vi "Follow Tilt.vi"(4 "L/T":bool, 6 "deg":i16, 8 "In":u8[][](array[numeric])) -> (0 "Out":u8[][](array[numeric]))   [LabVIEW 2015]
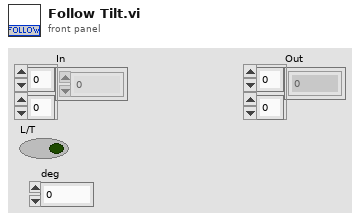
[diagram p1: front panel]
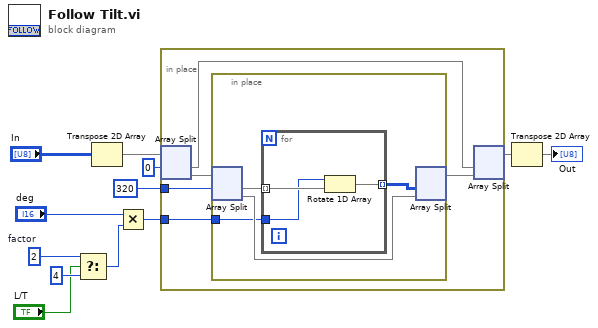
[diagram p0: block diagram]
diagram:
  w4 = i16 2  # factor
  n1 = Select(t=w4, s="L/T", f=i16 4) -> (s? t:f=w3:i16)
  n2 = Transpose 2D Array(2D array="In") -> (transposed array=w8:u8[][])
  n3 = Multiply(x="deg", y=w3) -> (x*y=w7:i16)
  n4 = in-place {
    in-place-border: 320 ("length") -> [w15]
    in-place-border: w7 -> [w13]
    n5 = in-place-split #1(w8, 0 ("start")) -> (w17:u8[][], w14:u8[][])
    n6 = in-place {
      in-place-border: w13 -> [w18]
      n7 = in-place-split #2(w14, w15) -> (w21:u8[][], w20:u8[][])
      n8 = for {
        tunnel: w21 -> [w24] mode=indexing
        tunnel: [w23] -> w19 mode=indexing
        tunnel: w18 -> [w22]
        n9 = Rotate 1D Array(1:w24, 2:w22) -> (0:w23:u8[])
      }
      n10 = in-place-split #2(w19, w20) -> (w16:u8[][])  [unwired: 1 out]
    }
    n11 = in-place-split #1(w17, w16) -> (w9:u8[][])  [unwired: 1 out]
  }
  n12 = Transpose 2D Array(2D array=w9) -> (transposed array=→"Out":u8[][])
